vi "Remove Image Outliers (I16).vi"(8 "error in (no error)":errorcluster, 9 "Percentile (0-100, Default: ignore)":dbl min=0.0 max=100.0, 10 "Delta (Default: ignore)":i16=32767, 11 "Data Value Reference in":refnum<data-value>) -> (0 "error out":errorcluster)   [LabVIEW 2021]
uses:
  57511ab9-796c-45ba-9bc9-c096f83d08ba.vi
  1b29086b-f2cd-41fe-a1ed-fdfc52a4aa66.vi
  d1a05142-2eb0-42fd-8c60-0af6ab015c0b.vi
  1fcef20d-819d-4864-a32f-c54cd922d116.vi
  d1a05142-2eb0-42fd-8c60-0af6ab015c0b.vi/3663a709-d1bc-4b7c-975a-3a90df5366f4.vi
  <vilib>/Comparison/Less/Less Functor/Less Functor.lvclass
panel:
  out "CPU (s)":dbl
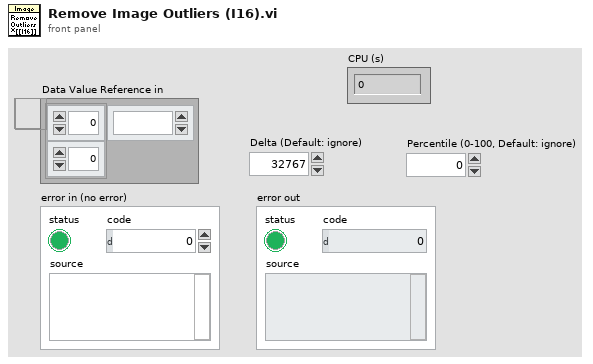
[diagram p1: front panel]
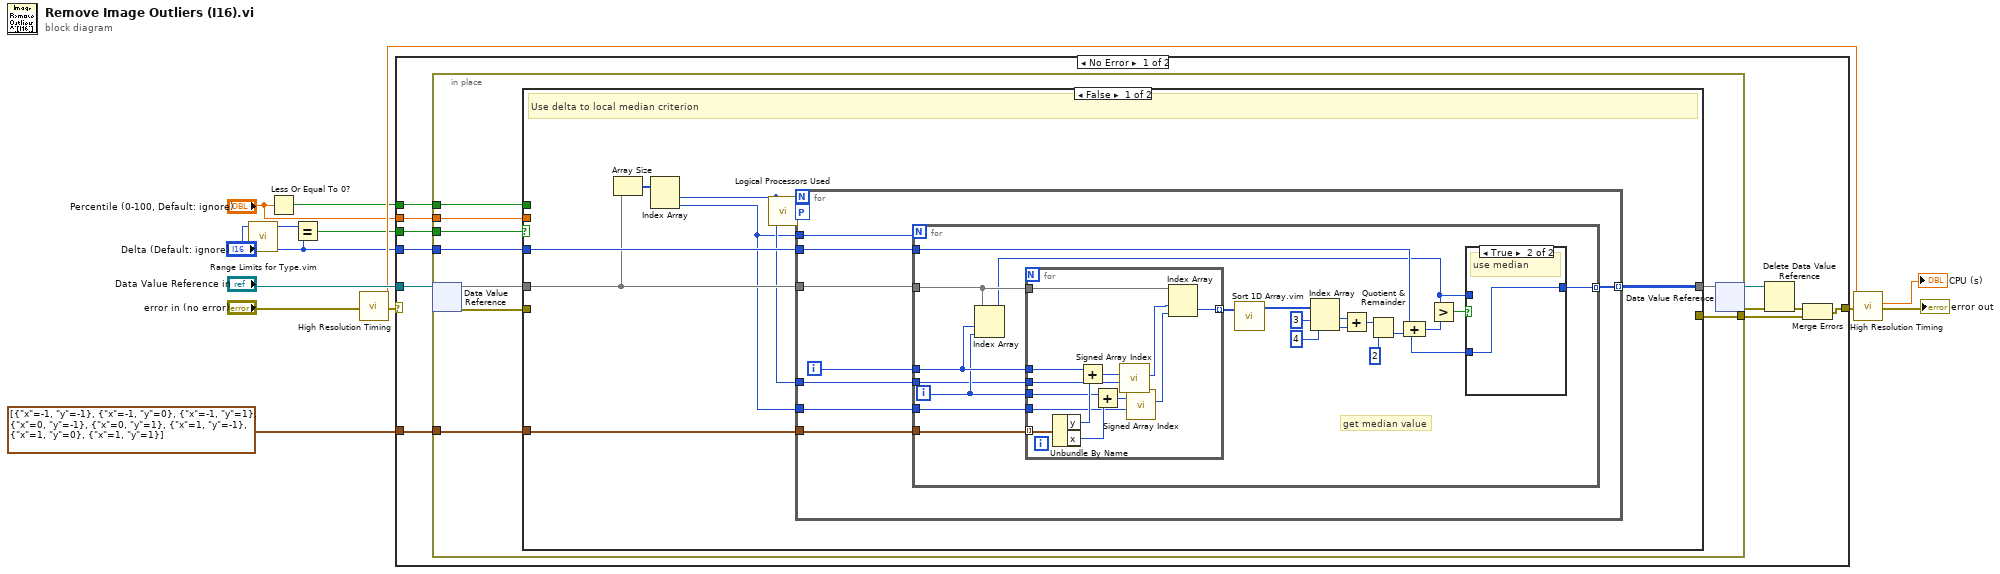
[diagram p0: block diagram]
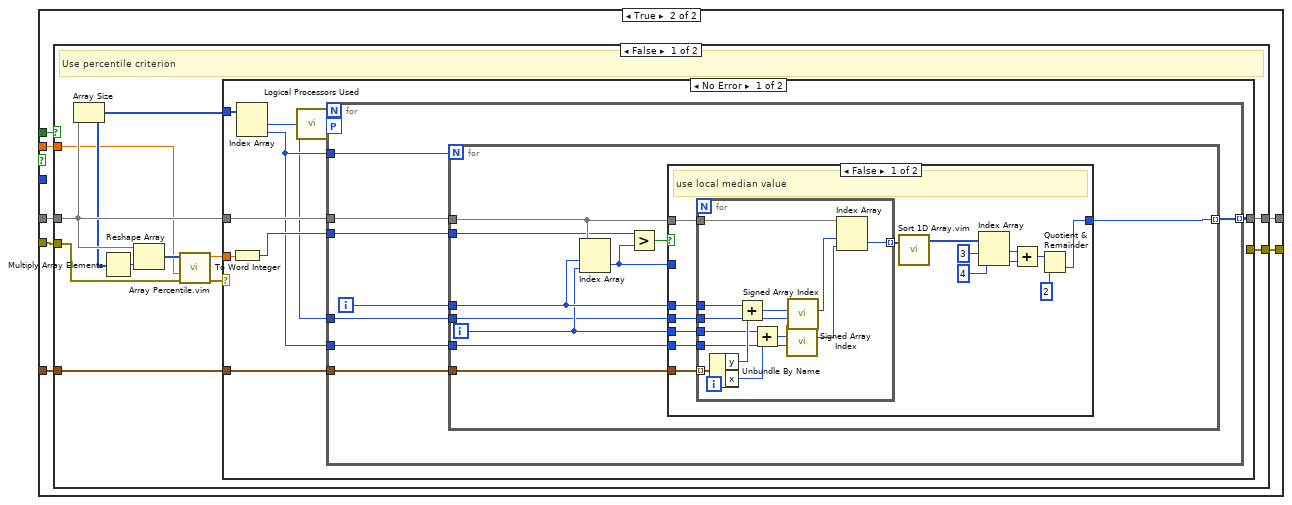
[diagram p3: hidden frame]
diagram:
  n1 = call "Range Limits for Type.vim"("type"="Delta (Default: ignore)") -> ("maximum value for type"=w5:i16)  [unwired: 9 in, 1 out]
  n2 = Less Or Equal To 0?(x="Percentile (0-100, Default: ignore)") -> (x <= 0?=w2:bool)
  n3 = Equal?(x=w5, y="Delta (Default: ignore)") -> (x = y?=w3:bool)
  n4 = call "High Resolution Timing.vi"("Error In"="error in (no error)") -> ("elapsed (relative) seconds"=w7:dbl, "Error Out"=w9:errorcluster)  [unwired: 16 in, 1 out]
  n5 = case shown="No Error" w9 {
    selector: w9 -> [_ w162]
    tunnel: "Data Value Reference in" -> [w24 _]
    tunnel: [w15 w162] -> w12
    tunnel: cluster{"x":i32, "y":i32}[] [{"x"=-1, "y"=-1}, {"x"=-1, "y"=0}, {"x"=-1, "y"=1}, {"x"=0, "y"=-1}, {"x"=0, "y"=1}, {"x"=1, "y"=-1}, {"x"=1, "y"=0}, {"x"=1, "y"=1}] -> [w20 _]
    tunnel: "Delta (Default: ignore)" -> [w19 _]
    tunnel: w3 -> [w18 _]
    tunnel: w2 -> [w17 _]
    tunnel: "Percentile (0-100, Default: ignore)" -> [w16 _]
    frame No Error {
      n6 = in-place {
        in-place-border: w20 -> [w32]
        in-place-border: w19 -> [w31]
        in-place-border: w18 -> [w29]
        in-place-border: w17 -> [w28]
        in-place-border: w16 -> [w27]
        in-place-border: [w25] -> w14
        n7 = in-place-dvr #1(w24) -> (w33:i16[][], w26:errorcluster)
        n8 = case shown="False" w29 {
          tunnel: w33 -> [w38 w89]
          tunnel: w32 -> [w41 w91]
          tunnel: w31 -> [w40 _]
          tunnel: [w39 w90] -> w30
          tunnel: w28 -> [_ w88]
          tunnel: w27 -> [_ w85]
          tunnel: w26 -> [_ w87]
          tunnel: [_ w86] -> w25
          frame False {
            # "Use delta to local median criterion"
            n9 = Array Size(array=w38) -> (size(s)=w37:i32[])
            n10 = Index Array(array=w37) -> (element #1=w36:i32, element #2=w35:i32)  [unwired: 2 in]
            n11 = call "Logical Processors Used.vi"() -> ("# Logical Processor Used"=w34:i32)  [unwired: 6 in]
            n12 = for {
              N: w36 -> [_]
              tunnel: w38 -> [w49]
              tunnel: w41 -> [w48]
              tunnel: w40 -> [w47]
              tunnel: [w46] -> w39 mode=indexing
              tunnel: w35 -> [w45]
              tunnel: w36 -> [w43]
              tunnel: w35 -> [w42]
              workers-P: w34 -> [_]
              i -> [w44]
              n13 = for {
                N: w45 -> [_]
                tunnel: w44 -> [w67]
                tunnel: w49 -> [w68]
                tunnel: w48 -> [w69]
                tunnel: w47 -> [w66]
                tunnel: [w65] -> w46 mode=indexing
                tunnel: w43 -> [w51]
                tunnel: w42 -> [w50]
                i -> [w64]
                # "get median value"
                n14 = Index Array(array=w68, index (row)=w67, index (col)=w64) -> (element=w52:i16)
                n15 = for {
                  tunnel: w68 -> [w77]
                  tunnel: w69 -> [w82] mode=indexing
                  tunnel: w67 -> [w81]
                  tunnel: w64 -> [w79]
                  tunnel: [w76] -> w63 mode=indexing
                  tunnel: w51 -> [w71]
                  tunnel: w50 -> [w70]
                  n16 = Unbundle By Name(w82) -> ("y"=w80:i32, "x"=w78:i32)
                  n17 = Add(x=w81, y=w80) -> (x+y=w73:i32)
                  n18 = Add(x=w79, y=w78) -> (x+y=w75:i32)
                  n19 = call "Signed Array Index.vi"("Array Size"=w71, "Array Index in"=w73) -> ("Array Index out"=w72:i32)  [unwired: 9 in]
                  n20 = call "Signed Array Index.vi"("Array Size"=w70, "Array Index in"=w75) -> ("Array Index out"=w74:i32)  [unwired: 9 in]
                  n21 = Index Array(array=w77, index (row)=w72, index (col)=w74) -> (element=w76:i16)
                }
                n22 = call "Sort 1D Array.vim"("unsorted array"=w63) -> ("sorted array"=w62:i16[])  [unwired: 10 in]
                n23 = Index Array(array=w62, index #1=3 ("index"), index #2=4 ("index")) -> (element #1=w59:i16, element #2=w58:i16)
                n24 = Add(x=w59, y=w58) -> (x+y=w57:i16)
                n25 = Quotient & Remainder(x=w57, y=i16 2) -> (floor(x/y)=w53:i16)  [unwired: 1 out]
                n26 = Compound Arithmetic op=ADD(w66, w53) -> (w55:i16)
                n27 = Greater?(x=w52, y=w55) -> (0:w54:bool)
                n28 = case shown="True" w54 {
                  tunnel: w53 -> [_ w84]
                  tunnel: w52 -> [w83 _]
                  tunnel: [w83 w84] -> w65
                  frame False {
                    # "keep"
                  }
                  frame True {
                    # "use median"
                  }
                }
              }
            }
          }
          frame True {
            n29 = case shown="False" w88 {
              tunnel: w91 -> [w102 _]
              tunnel: [w101 w161] -> w90
              tunnel: w89 -> [w98 w161]
              tunnel: w87 -> [w96 _]
              tunnel: [w94 _] -> w86
              tunnel: w85 -> [w92 _]
              frame False {
                # "Use percentile criterion"
                n30 = Array Size(array=w98) -> (size(s)=w97:i32[])
                n31 = Multiply Array Elements(1:w97) -> (0:w100:i32)
                n32 = Reshape Array(w98, w100) -> (w99:i16[])
                n33 = call "Array Percentile.vim"("Error In"=w96, "Percentile (0-100)"=w92, "Array"=w99) -> ("Error Out"=w95:errorcluster, "Percentile Value"=w93:dbl)  [unwired: 7 in]
                n34 = case shown="No Error" w95 {
                  selector: w95 -> [_ w159]
                  tunnel: w102 -> [w111 _]
                  tunnel: [w110 w160] -> w101
                  tunnel: w98 -> [w109 w160]
                  tunnel: w97 -> [w108 _]
                  tunnel: [_ w159] -> w94
                  tunnel: w93 -> [w107 _]
                  frame No Error {
                    n35 = To Word Integer(number=w107) -> (16bit integer=w106:i16)
                    n36 = Index Array(array=w108) -> (element #1=w104:i32, element #2=w105:i32)  [unwired: 2 in]
                    n37 = call "Logical Processors Used.vi"() -> ("# Logical Processor Used"=w103:i32)  [unwired: 6 in]
                    n38 = for {
                      N: w104 -> [_]
                      tunnel: w109 -> [w119]
                      tunnel: w111 -> [w118]
                      tunnel: [w117] -> w110 mode=indexing
                      tunnel: w105 -> [w116]
                      tunnel: w106 -> [w114]
                      tunnel: w105 -> [w113]
                      tunnel: w104 -> [w112]
                      workers-P: w103 -> [_]
                      i -> [w115]
                      n39 = for {
                        N: w116 -> [_]
                        tunnel: w115 -> [w127]
                        tunnel: w119 -> [w128]
                        tunnel: w118 -> [w129]
                        tunnel: [w126] -> w117 mode=indexing
                        tunnel: w114 -> [w124]
                        tunnel: w113 -> [w121]
                        tunnel: w112 -> [w120]
                        i -> [w125]
                        n40 = Index Array(array=w128, index (row)=w127, index (col)=w125) -> (element=w122:i16)
                        n41 = Greater?(x=w124, y=w122) -> (0:w123:bool)
                        n42 = case shown="False" w123 {
                          tunnel: w129 -> [w144 _]
                          tunnel: w128 -> [w135 _]
                          tunnel: w127 -> [w134 _]
                          tunnel: w125 -> [w133 _]
                          tunnel: [w132 w158] -> w126
                          tunnel: w122 -> [_ w158]
                          tunnel: w121 -> [w131 _]
                          tunnel: w120 -> [w130 _]
                          frame False {
                            # "use local median value"
                            n43 = for {
                              tunnel: w135 -> [w152]
                              tunnel: w144 -> [w157] mode=indexing
                              tunnel: w134 -> [w156]
                              tunnel: w133 -> [w154]
                              tunnel: [w151] -> w143 mode=indexing
                              tunnel: w131 -> [w146]
                              tunnel: w130 -> [w145]
                              n44 = Unbundle By Name(w157) -> ("y"=w155:i32, "x"=w153:i32)
                              n45 = Add(x=w156, y=w155) -> (x+y=w148:i32)
                              n46 = Add(x=w154, y=w153) -> (x+y=w150:i32)
                              n47 = call "Signed Array Index.vi"("Array Size"=w146, "Array Index in"=w150) -> ("Array Index out"=w149:i32)  [unwired: 9 in]
                              n48 = call "Signed Array Index.vi"("Array Size"=w145, "Array Index in"=w148) -> ("Array Index out"=w147:i32)  [unwired: 9 in]
                              n49 = Index Array(array=w152, index (row)=w147, index (col)=w149) -> (element=w151:i16)
                            }
                            n50 = call "Sort 1D Array.vim"("unsorted array"=w143) -> ("sorted array"=w142:i16[])  [unwired: 10 in]
                            n51 = Index Array(array=w142, index #1=3 ("index"), index #2=4 ("index")) -> (element #1=w139:i16, element #2=w138:i16)
                            n52 = Add(x=w139, y=w138) -> (x+y=w137:i16)
                            n53 = Quotient & Remainder(x=w137, y=i16 2) -> (floor(x/y)=w132:i16)  [unwired: 1 out]
                          }
                          frame True {
                            # "keep value"
                          }
                        }
                      }
                    }
                  }
                  frame Error {
                  }
                }
              }
              frame True {
                # "do nothing"
              }
            }
          }
        }
        n54 = in-place-dvr #1(w30) -> (w23:refnum<data-value>, w22:errorcluster)
      }
      n55 = Delete Data Value Reference(data value reference=w23, error in=w22) -> (error out=w21:errorcluster)  [unwired: 1 out]
      n56 = Merge Errors(w21, w14) -> (w15:errorcluster)
    }
    frame Error {
    }
  }
  n57 = call "High Resolution Timing.vi"("relative seconds (NaN)"=w7, "Error In"=w12) -> ("elapsed (relative) seconds"=→"CPU (s)":dbl, "Error Out"=→"error out":errorcluster)  [unwired: 15 in, 1 out]
